vi "CopyRawMemoryToImageGreyscale.vi"(8 "error in (no error)":errorcluster, 10 "Greyscale Destination Image":refnum<data-value>, 11 "Source":T1) -> (0 "error out":errorcluster, 3 "Greyscale Destination Image (duplicate)":refnum<data-value>)   [LabVIEW 2020, in "g_ar_toolkit.image.lvlib"]
uses:
  g_ar_toolkit.image.lvlib
  Raw Memory Information.ctl
  Raw Memory Information Dimension.ctl
  g_ar_toolkit.common/Module Path.vi
  <vilib>/Utility/error.llb/Error Cluster From Error Code.vi
  e0109ec8-11ee-4a07-aeee-d632e4e22c38.vi
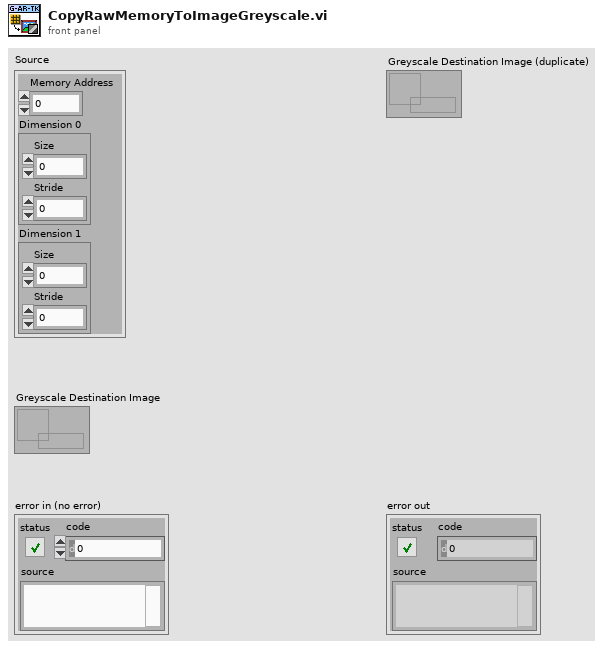
[diagram p1: front panel]
types:
  T1 = typedef "g_ar_toolkit.image.lvlib/Raw Memory Information.ctl" = cluster{"Memory Address":u64, "Dimension 0":T2, "Dimension 1":T2}
  T2 = typedef "g_ar_toolkit.image.lvlib/Raw Memory Information Dimension.ctl" = cluster{"Size":u16, "Stride":u32}
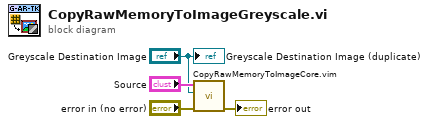
[diagram p0: block diagram]
diagram:
  n1 = call "CopyRawMemoryToImageCore.vim"("error in (no error)"="error in (no error)", "Dst"="Greyscale Destination Image", "Source"="Source") -> ("error out"=→"error out":errorcluster)  [unwired: 8 in]
  "Greyscale Destination Image (duplicate)" <- "Greyscale Destination Image"
